vi "Lambda Flow Auto (Set).vi"(6 "ISOBUS address":T2=-1 caption="ISOBUS address (-1)", 8 "error in":errorcluster, 10 "Lambda Auto":string, 11 "Mercury Reference In":T4) -> (0 "error out":errorcluster, 2 "Response":T1, 3 "Mercury Reference Out":T4, 4 "Valid?":T3)   [LabVIEW 2019, in "Mercury iXX.lvlib" / "Lambda.lvlib"]
doc: "Set the flow PID to be in automatic mode or manual."
uses:
  Lambda.lvlib
  Controls/Mercury Reference.ctl
  Controls/Comms Transport Layer.ctl
  Private/Controls/Query Dynamic Reference.ctl
  Controls/Is Valid LED.ctl
  Controls/ISOBus Address.ctl
  Controls/Response String.ctl
  Private/Controls/Command Verbs.ctl
  Mercury iXX.lvlib
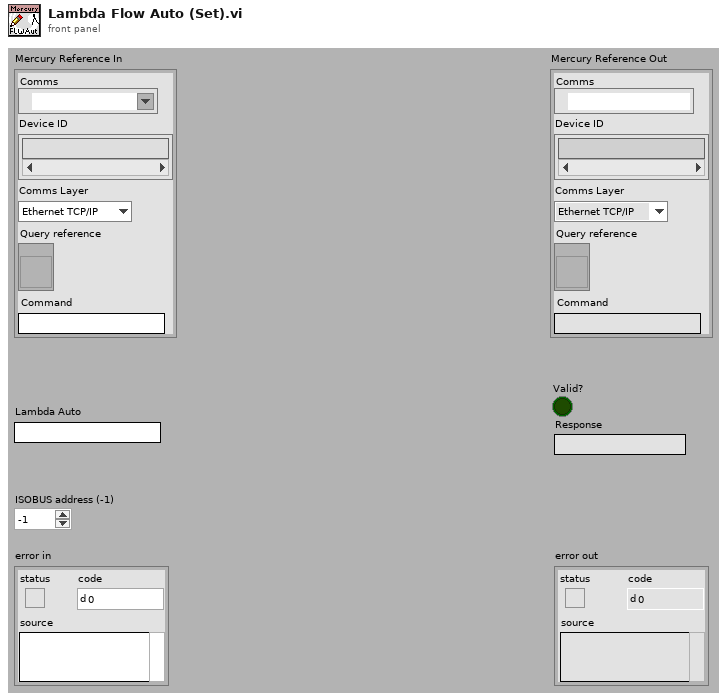
[diagram p1: front panel]
types:
  T1 = typedef "Mercury iXX.lvlib/Response String.ctl" = string
  T2 = typedef "Mercury iXX.lvlib/ISOBus Address.ctl" = i32
  T3 = typedef "Mercury iXX.lvlib/Is Valid LED.ctl" = bool
  T4 = typedef "Mercury iXX.lvlib/Mercury Reference.ctl" = cluster{"Comms":refnum<visa-resource-name>, "Device ID":string[], "Comms Layer":T5, "Command":string, "Query reference":T6}
  T5 = typedef "Mercury iXX.lvlib/Comms Transport Layer.ctl" = enum16{"Ethernet TCP/IP", "USB", "ISOBus - RS-232", "GPIB"}
  T6 = typedef "Mercury iXX.lvlib/Query Dynamic Reference.ctl" = refnum<vi>
  T7 = typedef "Mercury iXX.lvlib/Command Verbs.ctl" = string
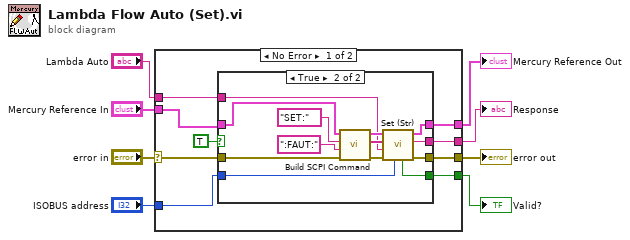
[diagram p0: block diagram]
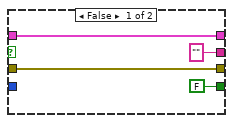
[diagram p2: hidden frame]
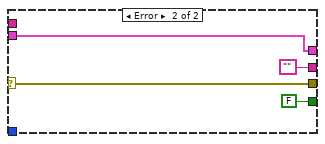
[diagram p3: hidden frame]
diagram:
  n1 = case shown="No Error" "error in" {
    selector: "error in" -> [w9 w37]
    tunnel: "Mercury Reference In" -> [w10 w38]
    tunnel: [w16 w38] -> w6
    tunnel: [w15 w37] -> w3
    tunnel: "ISOBUS address" -> [w17 _]
    tunnel: [w14 ""] -> w5
    tunnel: [w13 FALSE ("Valid?")] -> w4
    tunnel: "Lambda Auto" -> [w12 _]
    frame No Error {
      n2 = case shown="True" TRUE {
        tunnel: w12 -> [_ w22]
        tunnel: w9 -> [w21 w23]
        tunnel: w17 -> [_ w24]
        tunnel: w10 -> [w20 w29]
        tunnel: [w20 w28] -> w16
        tunnel: [w21 w27] -> w15
        tunnel: [T1 "" ("Response") w26] -> w14
        tunnel: [T3 FALSE ("Valid?") w25] -> w13
        frame False {
        }
        frame True {
          n3 = call "Build SCPI Command.vi"("error in"=w23, "Noun(s)"=":FAUT:" ("Command"), "Verb"=T7 "SET:", "Mercury Reference In"=w29) -> ("error out"=w34:errorcluster, "SCPI Message(s)"=w33:string[], "Mercury Reference Out"=w32:T4)  [unwired: 5 out]
          n4 = call "Set (Str).vi"("ISOBUS address"=w24, "error in"=w34, "Command Value (Str)"=w22, "SCPI Message(s)"=w33, "Mercury Reference In"=w32) -> ("error out"=w27:errorcluster, "Response"=w26:T1, "Mercury Reference Out"=w28:T4, "Valid?"=w25:T3)  [unwired: 3 out]
        }
      }
    }
    frame Error {
    }
  }
  "Mercury Reference Out" <- w6
  "error out" <- w3
  "Valid?" <- w4
  "Response" <- w5
